vi "SRV_Sensor PARSE_##iN.vi"(0 "Return Data":string) -> (3 "Sensor View Indicator Names":T1, 10 "Value":u16)   [LabVIEW 2014]
uses:
  SRV_Sensors Names.ctl
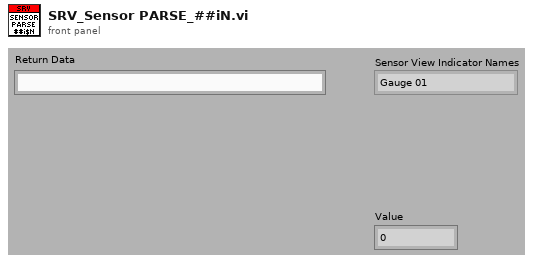
[diagram p1: front panel]
types:
  T1 = typedef "SRV_Sensors Names.ctl" = enum16{"Gauge 01", "Gauge 02", "Gauge 03", "Gauge 04", "Meter 01", "Meter 02", "Meter 03", "Meter 04", "Numeric 01", "Numeric 02", "Numeric 03", "Numeric 04", "Numeric 05", "Numeric 06", "Numeric 07", "Numeric 08", "Boolean 01", "Boolean 02", "Boolean 03", "Boolean 04", "Boolean 05", "Boolean 06", "Boolean 07", "Boolean 08", "Boolean 09", "Boolean 10", "Boolean 11", "Boolean 12", "Boolean 13", "Boolean 14", "Boolean 15", "Boolean 16", "Boolean 17", "Boolean 18", "Boolean 19", "Boolean 20", "Boolean 21", "Boolean 22", "Boolean 23", "Boolean 24", "Boolean 25", "Boolean 26", "Boolean 27", "Boolean 28", "Boolean 29", "Boolean 30", "Boolean 31", "Boolean 32"}
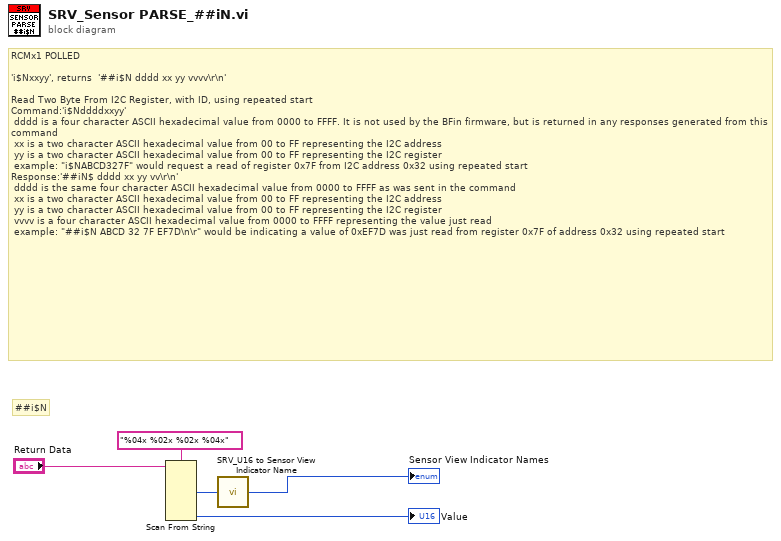
[diagram p0: block diagram]
diagram:
  # "##i$N"
  # "RCMx1 POLLED\n\n'i$Nxxyy', returns  '##i$N dddd xx yy vvvv\\r\\n'\n\nRead Two Byte From I2C Register, with ID, using repeated start\nCommand:'i$Nddddxxyy'\n dddd is a four character ASCII hexadecimal value from 0000 to FFFF. It is not used by the BFin firmware, but is returned in any responses generated from this command\n xx is a two character ASCII hexadecimal value from 00 to FF representing the I2C address\n yy is a two character ASCII hexadecimal value from 00 to FF representing the I2C register\n example: \"i$NABCD327F\" would request a read of register 0x7F from I2C address 0x32 using repeated start\nResponse:'##iN$ dddd xx yy vv\\r\\n'\n dddd is the same four character ASCII hexadecimal value from 0000 to FFFF as was sent in the command\n xx is a two character ASCII hexadecimal value from 00 to FF representing the I2C address\n yy is a two character ASCII hexadecimal value from 00 to FF representing the I2C register\n vvvv is a four character ASCII hexadecimal value from 0000 to FFFF representing the value just read\n example: \"##i$N ABCD 32 7F EF7D\\n\\r\" would be indicating a value of 0xEF7D was just read from register 0x7F of address 0x32 using repeated start"
  n1 = Scan From String(format string="%04x %02x %02x %04x", input string="Return Data") -> (output 1=w4:u32, output 4=→"Value":u16)  [unwired: 8 in, 3 out]
  n2 = call "SRV_U16 to Sensor View Indicator Name.vi"("U16"=w4) -> ("Sensor View Indicator Names"=→"Sensor View Indicator Names":T1)  [unwired: 14 in]
